vi "Pulse - Calculate Pulse_SubVI.vi"(10 "New Pulse Data":dbl[](array[numeric]), 11 "Existing Pulse Data":dbl[](array[numeric])) -> (1 "# found":i32, 2 "Heart Rate":dbl, 3 "Pulse Array Out":dbl[](array[numeric]))   [LabVIEW 2021]
uses:
  <vilib>/Analysis/3filter.llb/Filter Passband Type.ctl
  <vilib>/Analysis/3filter.llb/Butterworth Filter (DBL).vi
  <vilib>/Analysis/NI_AALBase.lvlib
  <vilib>/Analysis/NI_AAL_SigProc.lvlib
panel:
  out "size(s)":i32
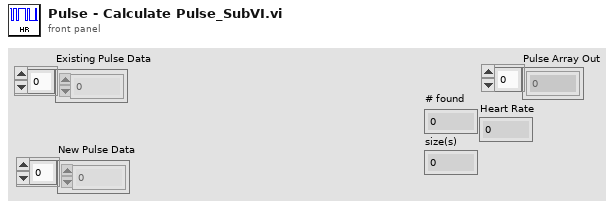
[diagram p1: front panel]
types:
  T1 = typedef "NI_AALBase.lvlib/Filter Passband Type.ctl" = enum32{"Lowpass", "Highpass", "Bandpass", "Bandstop"}
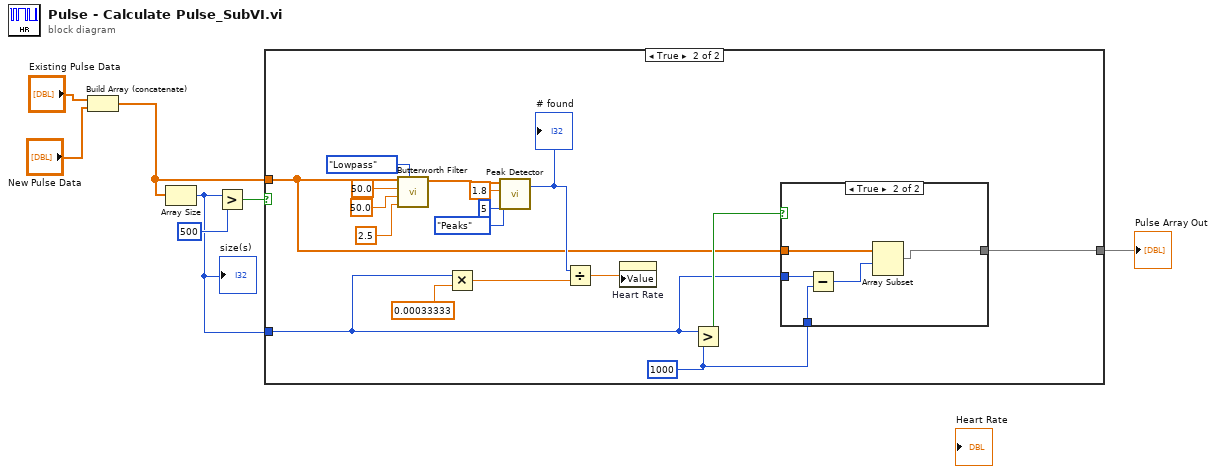
[diagram p0: block diagram]
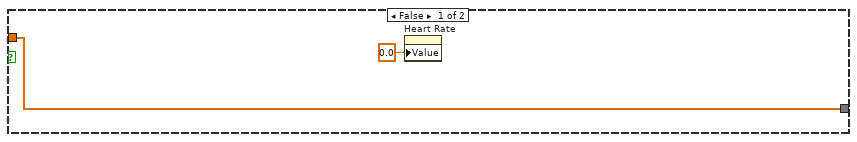
[diagram p2: hidden frame]
diagram:
  n1 = Build Array (concatenate)("Existing Pulse Data", "New Pulse Data") -> (w1:dbl[])
  n2 = Array Size(array=w1) -> (size(s)=w5:i32)
  "size(s)" <- w5
  n3 = Greater?(x=w5, y=500) -> (0:w6:bool)
  n4 = case shown="True" w6 {
    tunnel: w5 -> [_ w12]
    tunnel: w1 -> [w9 w14]
    tunnel: [w9 w13] -> w4
    frame False {
      n5 = property on="Heart Rate" class="DigNum (strict)"("Value"=0.0 ("Heart Rate")) -> ()  [unwired: 2 in, 2 out]
    }
    frame True {
      w11 = 1000 ("y")
      n6 = call-poly <vilib>:"Butterworth Filter.vi"("filter type"=Filter_Passband_Type."Lowpass", "low cutoff freq: fl"=2.5, "high cutoff freq: fh"=50.0, "sampling freq: fs"=50.0, "X"=w14) -> ("Filtered X"=w22:dbl[])  [unwired: 3 in, 1 out]
      n7 = Multiply(x=w12, y=0.00033333) -> (x*y=w17:dbl)
      n8 = call <vilib>:"Peak Detector.vi"("peaks/valleys"=enum32{"Peaks", "Valleys"}."Peaks", "width"=5, "threshold"=1.8, "X"=w22) -> ("# found"=w18:i32)  [unwired: 3 in, 4 out]
      "# found" <- w18
      n9 = Divide(x=w18, y=w17) -> (x/y=w10:dbl)
      n10 = property on="Heart Rate" class="DigNum (strict)"("Value"=w10) -> ()  [unwired: 2 in, 2 out]
      n11 = Greater?(x=w12, y=w11) -> (0:w15:bool)
      n12 = case shown="True" w15 {
        tunnel: w14 -> [w27 w32]
        tunnel: [w27 w28] -> w13
        tunnel: w12 -> [_ w31]
        tunnel: w11 -> [_ w30]
        frame False {
        }
        frame True {
          n13 = Subtract(x=w31, y=w30) -> (x-y=w29:i32)
          n14 = Array Subset(array=w32, index=w29) -> (w28:dbl[])  [unwired: 1 in]
        }
      }
    }
  }
  "Pulse Array Out" <- w4
